vi "Tosca-Process Message.vi"(0 "Progress In":T2, 5 "Message":refnum<queue>, 7 "timeout in ms":i32, 9 "State":i32, 11 "error in (no error)":errorcluster) -> (4 "Progress Out":T2, 8 "Action":T1, 15 "error out":errorcluster)   [LabVIEW 2020]
uses:
  IPC VIs/Tosca-Message.ctl
  IPC VIs/Tosca-Message Action.ctl
  Typedefs/Tosca-Transition Progress.ctl
  Typedefs/Tosca-Trial Result Enum.ctl
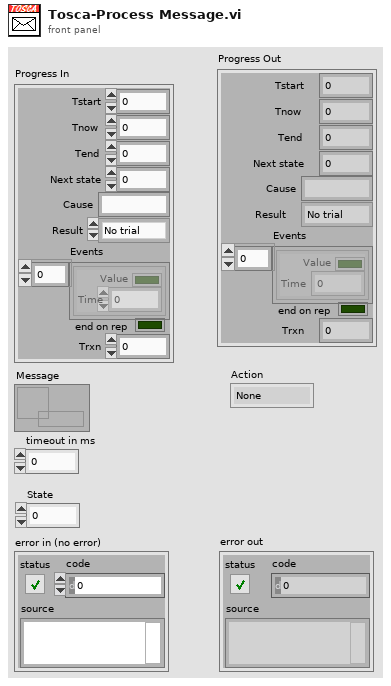
[diagram p1: front panel]
types:
  T1 = typedef "Tosca-Message Action.ctl" = enum16{"None", "Update", "Events", "Timeout", "Error", "Abort"}
  T2 = typedef "Tosca-Transition Progress.ctl" = cluster{"Tstart":u32, "Tnow":u32, "Tend":dbl, "Next state":i32, "Cause":string, "Result":T3, "Events":cluster{"Value":bool, "Time":u32}[], "end on rep":bool, "Trxn":i32}
  T3 = typedef "Tosca-Trial Result Enum.ctl" = enum16{"No trial", "Go", "No go", "Error", "Abort"}
  T4 = typedef "Tosca-Message.ctl" = cluster{"Action":T1, "Time":u32, "State":i32, "Events":bool[], "Error":errorcluster}
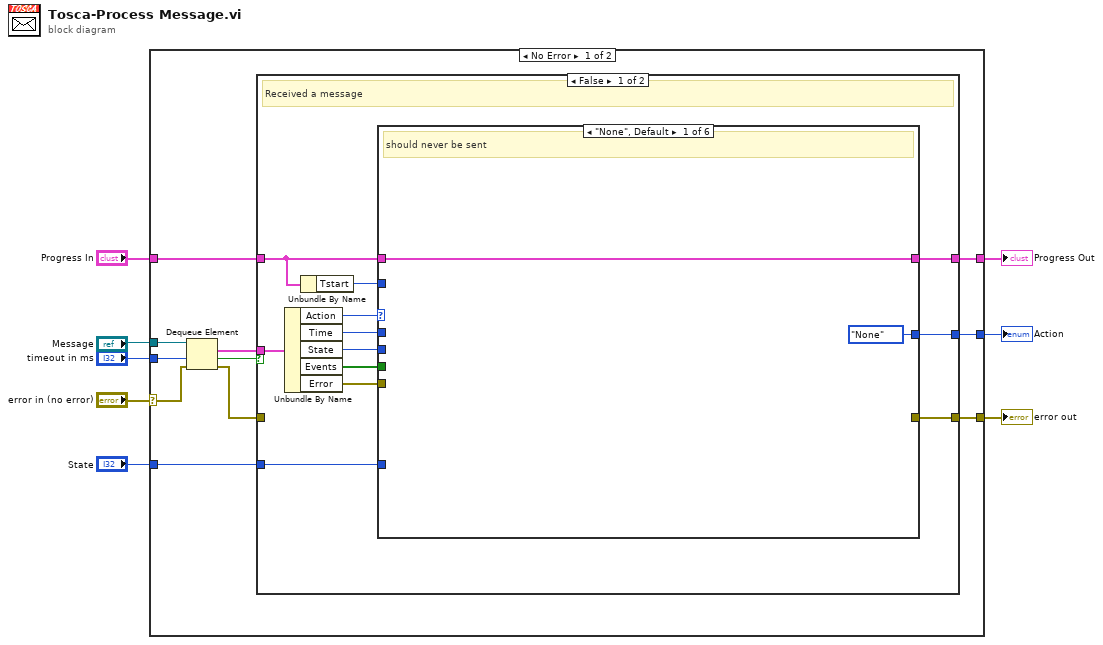
[diagram p0: block diagram]
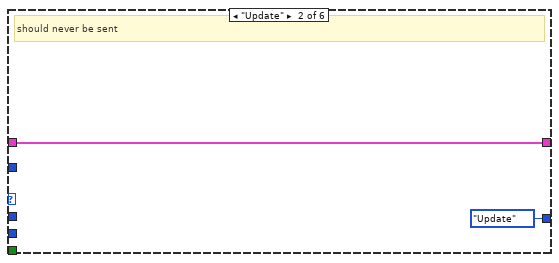
[diagram p2: hidden frame]
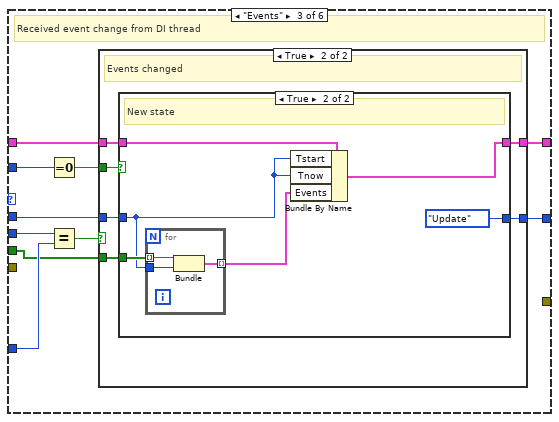
[diagram p3: hidden frame]
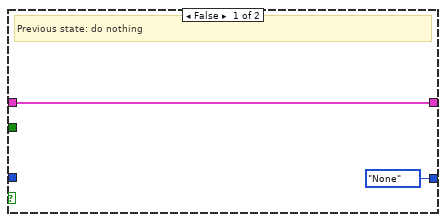
[diagram p4: hidden frame]
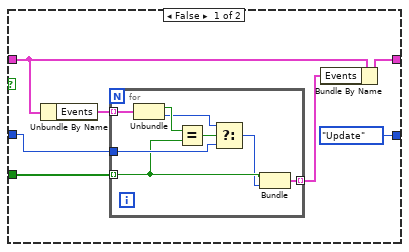
[diagram p5: hidden frame]
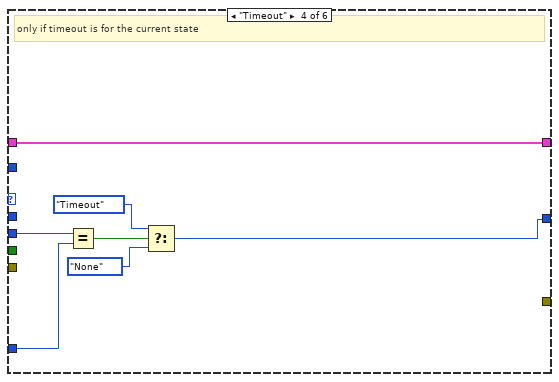
[diagram p6: hidden frame]
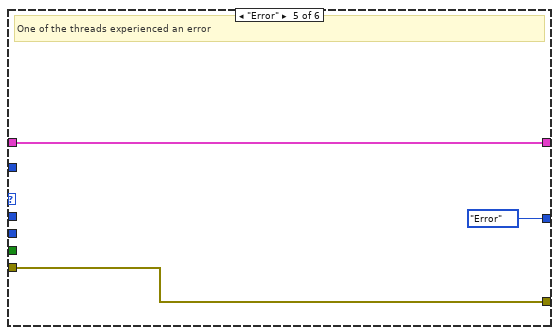
[diagram p7: hidden frame]
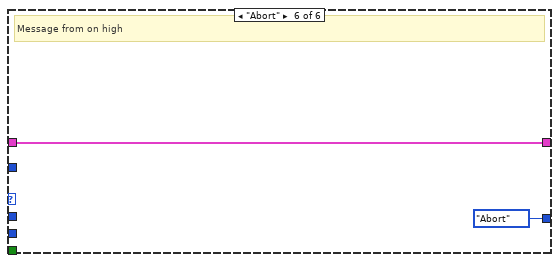
[diagram p8: hidden frame]
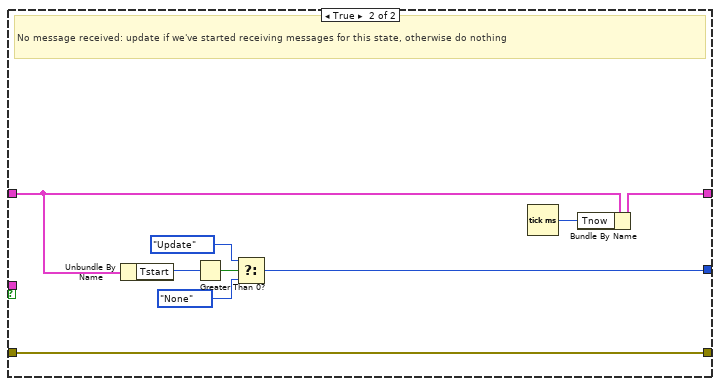
[diagram p9: hidden frame]
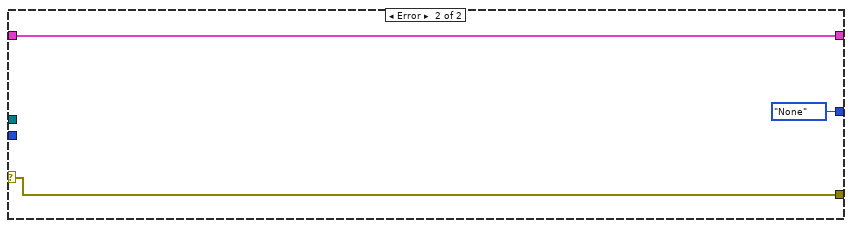
[diagram p10: hidden frame]
diagram:
  n1 = case shown="No Error" "error in (no error)" {
    selector: "error in (no error)" -> [w16 w100]
    tunnel: "timeout in ms" -> [w19 _]
    tunnel: "Message" -> [w18 _]
    tunnel: "Progress In" -> [w13 w101]
    tunnel: [w12 w101] -> w4
    tunnel: [w11 Tosca-Message_Action."None" ("Action")] -> w3
    tunnel: [w10 w100] -> w2
    tunnel: "State" -> [w9 _]
    frame No Error {
      n2 = Dequeue Element(queue=w18, timeout in ms (-1)=w19, error in (no error)=w16) -> (element=w15:T4, timed out?=w17:bool, error out=w14:errorcluster)  [unwired: 1 out]
      n3 = case shown="False" w17 {
        tunnel: w15 -> [w31 _]
        tunnel: [w28 w92] -> w10
        tunnel: w14 -> [_ w92]
        tunnel: w13 -> [w21 w93]
        tunnel: [w24 w94] -> w11
        tunnel: [w23 w91] -> w12
        tunnel: w9 -> [w22 _]
        frame False {
          # "Received a message"
          n4 = Unbundle By Name(w31) -> ("Action"=w30:T1, "Time"=w27:u32, "State"=w26:i32, "Events"=w25:bool[], "Error"=w29:errorcluster)
          n5 = Unbundle By Name(w21) -> ("Tstart"=w20:u32)
          n6 = case shown="\"None\", Default" w30 {
            tunnel: w29 -> [_ _ _ _ w87 _]
            tunnel: [_ _ _ _ w87 _] -> w28
            tunnel: w27 -> [_ _ w37 _ _ _]
            tunnel: w26 -> [_ _ w45 w83 _ _]
            tunnel: w25 -> [_ _ w38 _ _ _]
            tunnel: [Tosca-Message_Action."None" ("Action") Tosca-Message_Action."Update" ("Action") w40 w78 Tosca-Message_Action."Error" ("Action") Tosca-Message_Action."Abort" ("Action")] -> w24
            tunnel: w21 -> [w32 w34 w43 w84 w86 w88]
            tunnel: [w32 w34 w42 w84 w86 w88] -> w23
            tunnel: w22 -> [_ _ w44 w82 _ _]
            tunnel: w20 -> [_ _ w36 _ _ _]
            frame "None", Default {
              # "should never be sent"
            }
            frame "Update" {
              # "should never be sent"
            }
            frame "Events" {
              # "Received event change from DI thread"
              n7 = Equal To 0?(x=w36) -> (x = 0?=w39:bool)
              n8 = Equal?(x=w45, y=w44) -> (x = y?=w41:bool)
              n9 = case shown="True" w41 {
                tunnel: w43 -> [w47 w52]
                tunnel: [w47 w51] -> w42
                tunnel: [Tosca-Message_Action."None" ("Action") w48] -> w40
                tunnel: w39 -> [_ w53]
                tunnel: w37 -> [_ w50]
                tunnel: w38 -> [_ w49]
                frame False {
                  # "Previous state: do nothing"
                }
                frame True {
                  # "Events changed"
                  n10 = case shown="True" w53 {
                    tunnel: w52 -> [w60 w74]
                    tunnel: [w56 w73] -> w51
                    tunnel: w50 -> [w57 w71]
                    tunnel: w49 -> [w58 w72]
                    tunnel: [Tosca-Message_Action."Update" ("Action") Tosca-Message_Action."Update" ("Action")] -> w48
                    frame False {
                      n11 = Unbundle By Name(w60) -> ("Events"=w59:cluster{"Value":bool, "Time":u32}[])
                      n12 = for {
                        tunnel: w59 -> [w68] mode=indexing
                        tunnel: w58 -> [w63] mode=indexing
                        tunnel: w57 -> [w64]
                        tunnel: [w61] -> w55 mode=indexing
                        n13 = Unbundle(w68) -> ("Value"=w67:bool, "Time"=w65:u32)
                        n14 = Equal?(x=w67, y=w63) -> (x = y?=w66:bool)
                        n15 = Select(t=w65, s=w66, f=w64) -> (s? t:f=w62:u32)
                        n16 = Bundle("Boolean"=w63, "Time"=w62) -> (w61:cluster{"Boolean":bool, "Time":u32})  [unwired: 1 in]
                      }
                      n17 = Bundle By Name(cluster=w60, "Events"=w55) -> (w56:T2)
                    }
                    frame True {
                      # "New state"
                      n18 = for {
                        tunnel: w72 -> [w77] mode=indexing
                        tunnel: w71 -> [w76]
                        tunnel: [w75] -> w70 mode=indexing
                        n19 = Bundle("Boolean"=w77, "Time"=w76) -> (w75:cluster{"Boolean":bool, "Time":u32})  [unwired: 1 in]
                      }
                      n20 = Bundle By Name(cluster=w74, "Tstart"=w71, "Tnow"=w71, "Events"=w70) -> (w73:T2)
                    }
                  }
                }
              }
            }
            frame "Timeout" {
              # "only if timeout is for the current state"
              n21 = Equal?(x=w83, y=w82) -> (x = y?=w81:bool)
              n22 = Select(t=Tosca-Message_Action."Timeout" ("Action"), s=w81, f=Tosca-Message_Action."None") -> (s? t:f=w78:T1)
            }
            frame "Error" {
              # "One of the threads experienced an error"
            }
            frame "Abort" {
              # "Message from on high"
            }
          }
        }
        frame True {
          # "No message received: update if we've started receiving messages for this state, otherwise do nothing"
          n23 = Unbundle By Name(w93) -> ("Tstart"=w98:u32)
          n24 = Greater Than 0?(x=w98) -> (x > 0?=w97:bool)
          n25 = Select(t=Tosca-Message_Action."Update", s=w97, f=Tosca-Message_Action."None" ("Action")) -> (s? t:f=w94:T1)
          n26 = Tick Count (ms)() -> (millisecond timer value=w90:u32)
          n27 = Bundle By Name(cluster=w93, "Tnow"=w90) -> (w91:T2)
        }
      }
    }
    frame Error {
    }
  }
  "Progress Out" <- w4
  "error out" <- w2
  "Action" <- w3
